vi "Test.Maui 2.0.Initialize.Plenty.Rings.Ring 1.vi"(8 "error in":errorcluster) -> (0 "error out":errorcluster)   [LabVIEW 2019]
uses:
  Maui 2.0/Maui 2.0.lvclass
  <vilib>/JKI/JKI SMO/SMO/SMO.lvclass
  Helper/Test Helper 1/Test Helper 1.lvclass
  <vilib>/addons/_JKI Toolkits/Caraya/classes/Assert/Assert.lvclass
  <vilib>/addons/_JKI Toolkits/Caraya/classes/Assert/Assert Equal Value_Variant.vi
  <vilib>/addons/_JKI Toolkits/Caraya/classes/Test/Test.lvclass
  C:/Program Files (x86)/National Instruments/LabVIEW 2019/vi.lib/JKI/JKI SMO/SMO/SMO.lvclass
  <vilib>/addons/_JKI Toolkits/Caraya/classes/Assert/Assert True.vi
panel:
  in  "Ring 2":u16(ring) items=["Maui 2.0", "Test Helper 1", "Maui 2.0", "None"]
  in  "Ring":u16(ring) items=["Maui 2.0", "Test Helper 1", "Maui 2.0", "None"]
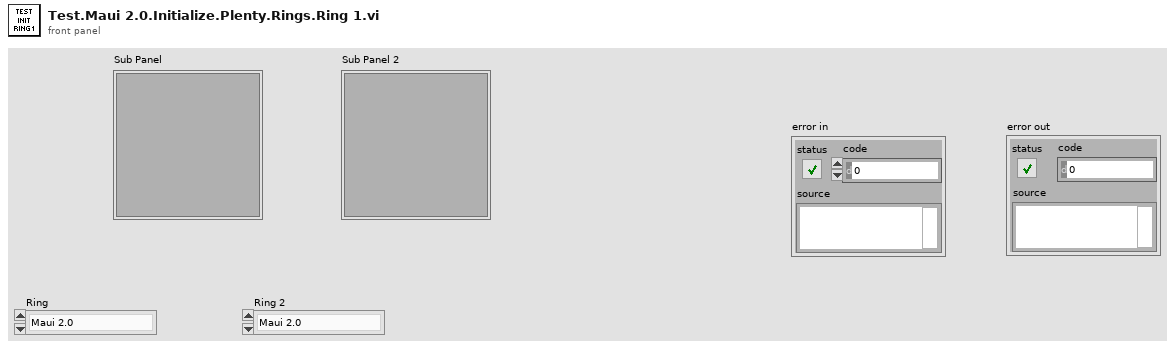
[diagram p1: front panel]
types:
  T1 = cluster{"Ring":refnum<vi>, "Sub Panel":refnum<vi>}
  T2 = cluster{"Ring 2":refnum<vi>, "Sub Panel 2":refnum<vi>}
  T3 = cluster{"Ring 2":refnum<vi>, "Sub Panel 2":refnum<vi>}[]
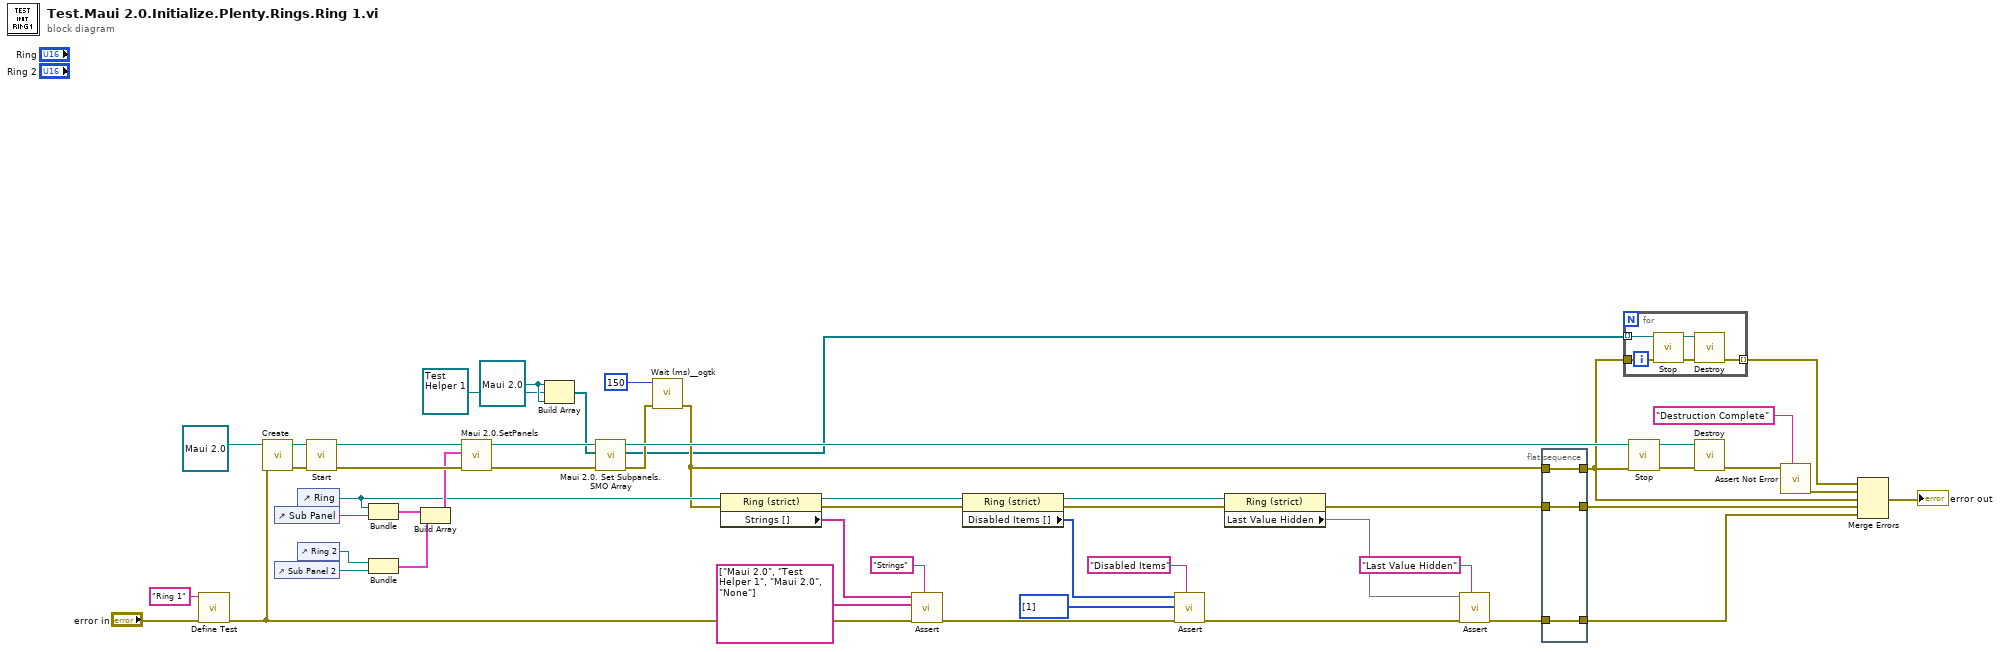
[diagram p0: block diagram]
diagram:
  w39 = refnum<class "Maui 2.0.lvclass"> refnum ("Maui 2.0 in")
  n1 = call <vilib>:"Define Test.vi"("error in (no error)"="error in", "Label (VI Title)"="Ring 1") -> ("error out"=w25:errorcluster)  [unwired: 9 in]
  n2 = call <vilib>:"Create.vi"("error in (no error)"=w25, "SMO"=refnum<class "Maui 2.0.lvclass"> refnum ("Maui 2.0 in")) -> ("error out"=w51:errorcluster, "SMO out"=w43:refnum<class "Maui 2.0.lvclass">)  [unwired: 7 in, 1 out]
  n3 = control-ref of="Sub Panel"() -> (w48:refnum<vi>)
  n4 = control-ref of="Sub Panel 2"() -> (w46:refnum<vi>)
  n5 = control-ref of="Ring"() -> (w35:refnum<vi>)
  n6 = control-ref of="Ring 2"() -> (w47:refnum<vi>)
  n7 = call <vilib>:"Start.vi"("error in (no error)"=w51, "SMO"=w43) -> ("error out"=w50:errorcluster, "SMO out"=w41:refnum<class "Maui 2.0.lvclass">)  [unwired: 8 in]
  n8 = Bundle("Ring"=w35, "Sub Panel"=w48) -> (w45:T1)  [unwired: 1 in]
  n9 = Bundle("Ring 2"=w47, "Sub Panel 2"=w46) -> (w44:T2)  [unwired: 1 in]
  n10 = Build Array(w45, w44) -> (w36:T3)
  n11 = call "Maui 2.0.SetPanels.vi"("error in (no error)"=w50, "Set Panels"=w36, "Maui 2.0"=w41) -> ("error out"=w49:errorcluster, "Maui 2.0 out"=w40:refnum<class "Maui 2.0.lvclass">)  [unwired: 7 in]
  n12 = Build Array(w39, refnum<class "Test Helper 1.lvclass"> refnum ("Test Helper 1.lvclass"), w39) -> (w37:refnum<class "SMO.lvclass">[])
  n13 = call-dynamic "Maui 2.0. Set Subpanels.SMO Array.vi"("error in (no error)"=w49, "Subpanels in"=w37, "Maui 2.0 in"=w40) -> ("error out"=w9:errorcluster, "Subpanels Out"=w6:refnum<class "SMO.lvclass">[], "Maui 2.0 out"=w19:refnum<class "Maui 2.0.lvclass">)  [unwired: 6 in]
  n14 = call <userlib>:"Wait (ms)__ogtk.vi"("error in (no error)"=w9, "milliseconds to wait"=u32 150) -> ("error out"=w8:errorcluster)  [unwired: 8 in, 1 out]
  n15 = property class="Ring (strict)"(reference=w35, error in=w8) -> (reference out=w29:refnum<vi>, error out=w22:errorcluster, "Strings []"=w33:string[])
  n16 = call-poly <vilib>:"Assert.vi"("Label"="Strings", "error in (no error)"=w25, "Y"=string[] ["Maui 2.0", "Test Helper 1", "Maui 2.0", "None"], "X"=w33) -> ("error out"=w23:errorcluster)  [unwired: 7 in]
  n17 = property class="Ring (strict)"(reference=w29, error in=w22) -> (reference out=w27:refnum<vi>, error out=w21:errorcluster, "Disabled Items []"=w3:i32[])
  n18 = call-poly <vilib>:"Assert.vi"("Label"="Disabled Items", "error in (no error)"=w23, "Y"=i32[] [1] ("Disabled Items []"), "X"=w3) -> ("error out"=w24:errorcluster)  [unwired: 7 in]
  n19 = property class="Ring (strict)"(reference=w27, error in=w21) -> (error out=w13:errorcluster, "Last Value Hidden"=w20)  [unwired: 1 out]
  n20 = call-poly <vilib>:"Assert.vi"("Label"="Last Value Hidden", "error in (no error)"=w24, "True?"=w20) -> ("error out"=w12:errorcluster)  [unwired: 8 in]
  n21 = flat-sequence {
    tunnel: w8 -> [w54]
    tunnel: w13 -> [w53]
    tunnel: w12 -> [w52]
    tunnel: [w54] -> w4
    tunnel: [w53] -> w11
    tunnel: [w52] -> w10
    frame #0 {
    }
  }
  n22 = for {
    tunnel: w6 -> [w58] mode=indexing
    tunnel: w4 -> [w57]
    tunnel: [w55] -> w5 mode=indexing
    n23 = call <vilib>:"Stop.vi"("error in (no error)"=w57, "SMO"=w58) -> ("error out"=w56:errorcluster, "SMO out"=w59:refnum<class "SMO.lvclass">)  [unwired: 8 in]
    n24 = call <vilib>:"Destroy.vi"("error in (no error)"=w56, "SMO"=w59) -> ("error out"=w55:errorcluster)  [unwired: 9 in]
  }
  n25 = call <vilib>:"Stop.vi"("error in (no error)"=w4, "SMO"=w19) -> ("error out"=w17:errorcluster, "SMO out"=w18:refnum<class "Maui 2.0.lvclass">)  [unwired: 8 in]
  n26 = call <vilib>:"Destroy.vi"("error in (no error)"=w17, "SMO"=w18) -> ("error out"=w16:errorcluster)  [unwired: 9 in]
  n27 = call <vilib>:"Assert Not Error.vi"("Label"="Destruction Complete", "Not Error?"=w16) -> ("error out"=w14:errorcluster)  [unwired: 9 in]
  n28 = Merge Errors(w5, w14, w4, w11, w10) -> (→"error out":errorcluster)
